vi "serialization.vi"() -> ()   [LabVIEW 2013, in "tag bus tests.lvlib"]
uses:
  tag bus tests.lvlib
  table/data table.ctl
  dictionary/data dictionary.lvclass/data dictionary.ctl
  dictionary/data dictionary.lvclass
  table/data table.lvlib
panel:
  out "e":string
  out "error out":errorcluster
  out "ok":bool
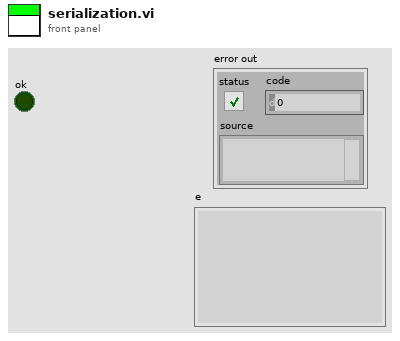
[diagram p1: front panel]
types:
  T1 = typedef "tag bus.lvlib/data table.lvlib/data table.ctl" = cluster{"Double":dbl[], "Single":sgl[], "I64":i64[], "I32":i32[], "I16":i16[], "I8":i8[], "U64":u64[], "U32":u32[], "U16":u16[], "U8":u8[], "Boolean":bool[], "String":string[], "Array of Double":cluster{"DBL Array":dbl[]}[], "Array of Single":cluster{"SGL Array":sgl[]}[], "Array of I64":cluster{"I64 Array":i64[]}[], "Array of I32":cluster{"I32 Array":i32[]}[], "Array of I16":cluster{"I16 Array":i16[]}[], "Array of I8":cluster{"I8 Array":i8[]}[], "Array of U64":cluster{"U64 Array":u64[]}[], "Array of U32":cluster{"U32 Array":u32[]}[], "Array of U16":cluster{"U16 Array":u16[]}[], "Array of U8":cluster{"U8 Array":u8[]}[], "Array of Boolean":cluster{"Boolean Array":bool[]}[], "Array of String":cluster{"String Array":string[]}[]}
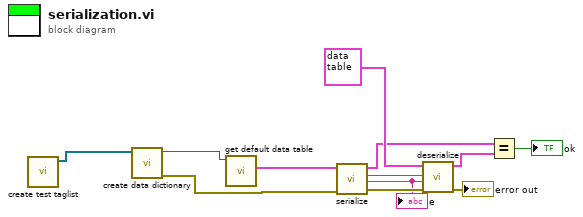
[diagram p0: block diagram]
diagram:
  n1 = call "create test taglist.vi"() -> ("tags"=w12:refnum<class "tag descriptor.lvclass">[])  [unwired: 8 in, 3 out]
  n2 = call "create data dictionary.vi"("system tags"=w12) -> ("error out"=w1:errorcluster, "data dictionary"=w11:refnum<class "data dictionary.lvclass">)  [unwired: 9 in]
  n3 = call "get default data table.vi"("data dictionary in"=w11) -> ("default data table"=w9:T1)  [unwired: 9 in, 1 out]
  n4 = call "serialize.vi"("error in"=w1, "data table in"=w9) -> ("error out"=w10:errorcluster, "data"=w7:string, "version"=w8:string, "data table out"=w4:T1)  [unwired: 6 in]
  "e" <- w7
  n5 = call "deserialize.vi"("error in"=w10, "data"=w7, "version"=w8, "data table in"=T1 {"Double"=[], "Single"=[], "I64"=[], "I32"=[], "I16"=[], "I8"=[], "U64"=[], "U32"=[], "U16"=[], "U8"=[], "Boolean"=[], "String"=[], "Array of Double"=[], "Array of Single"=[], "Array of I64"=[], "Array of I32"=[], "Array of I16"=[], "Array of I8"=[], "Array of U64"=[], "Array of U32"=[], "Array of U16"=[], "Array of U8"=[], "Array of Boolean"=[], "Array of String"=[]}) -> ("error out"=→"error out":errorcluster, "data table out"=w5:T1)  [unwired: 6 in]
  n6 = Equal?(x=w4, y=w5) -> (x = y?=→"ok":bool)
